vi "Wiring Colour.vi"() -> ()   [LabVIEW 2020]
panel:
  out "Boolean 2":bool
  in  "Boolean":bool
  out "String 2":string
  in  "String":string
  out "Numeric 4":i64
  in  "Numeric 3":i64
  out "Numeric 2":dbl
  in  "Numeric":dbl
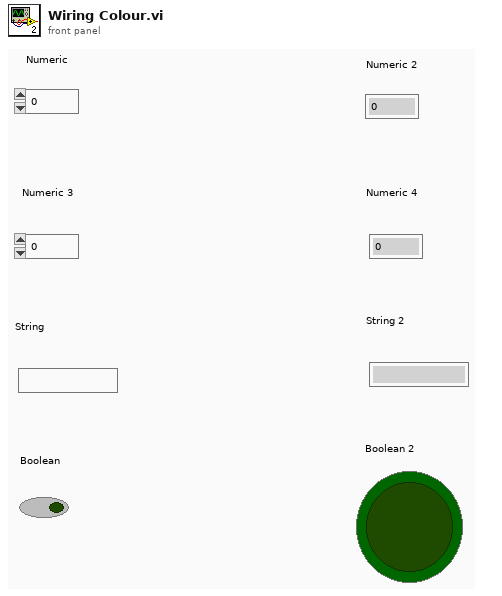
[diagram p1: front panel]
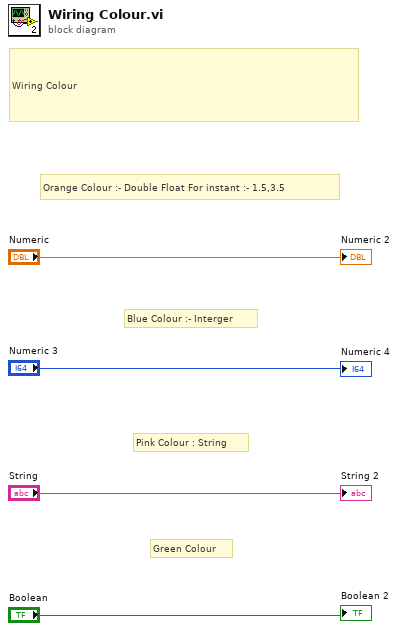
[diagram p0: block diagram]
diagram:
  # "Green Colour"
  # "Pink Colour : String"
  # "Blue Colour :- Interger"
  # "Orange Colour :- Double Float For instant :- 1.5,3.5"
  # "Wiring Colour"
  "Numeric 2" <- "Numeric"
  "Numeric 4" <- "Numeric 3"
  "String 2" <- "String"
  "Boolean 2" <- "Boolean"
